vi "Process Data Motor Init_vel.vi"(8 "에러 입력(에러 없음)":errorcluster) -> (0 "에러 출력":errorcluster)   [LabVIEW 2019]
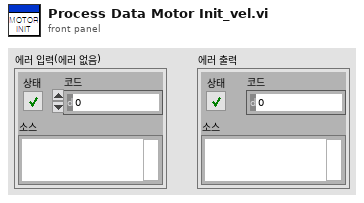
[diagram p1: front panel]
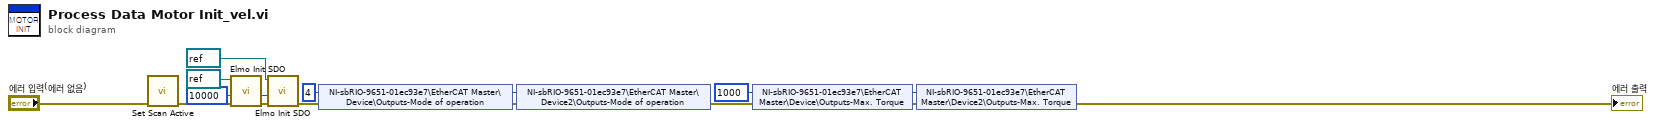
[diagram p0: block diagram]
diagram:
  w12 = u16 1000 ("Outputs-Max. Torque")
  w9 = i8 4 ("Outputs-Mode of operation")
  w5 = 10000 ("Timeout(Scans)")
  n1 = call "Set Scan Active.vi"("error in (no error)"="에러 입력(에러 없음)") -> ("Error Out"=w2:errorcluster)  [unwired: 10 in]
  n2 = call "Elmo Init SDO.vi"("Error In"=w2, "Timeout(Scans)"=w5, "Elmo Driver IO"=refnum<k21> "ni.var.io://ni-sbrio-9651-01ec93e7/EtherCAT Master/Device" ("Slave Constant")) -> ("error out"=w4:errorcluster)  [unwired: 8 in]
  n3 = call "Elmo Init SDO.vi"("Error In"=w4, "Timeout(Scans)"=w5, "Elmo Driver IO"=refnum<k21> "ni.var.io://ni-sbrio-9651-01ec93e7/EtherCAT Master/Device2" ("Slave Constant")) -> ("error out"=w7:errorcluster)  [unwired: 8 in]
  n4 = shared-variable "NI-sbRIO-9651-01ec93e7\\EtherCAT Master\\Device\\Outputs-Mode of operation"(w9, error in=w7) -> (error out=w8:errorcluster)
  n5 = shared-variable "NI-sbRIO-9651-01ec93e7\\EtherCAT Master\\Device2\\Outputs-Mode of operation"(w9, error in=w8) -> (error out=w10:errorcluster)
  n6 = shared-variable "NI-sbRIO-9651-01ec93e7\\EtherCAT Master\\Device\\Outputs-Max. Torque"(w12, error in=w10) -> (error out=w11:errorcluster)
  n7 = shared-variable "NI-sbRIO-9651-01ec93e7\\EtherCAT Master\\Device2\\Outputs-Max. Torque"(w12, error in=w11) -> (error out=→"에러 출력":errorcluster)
